vi "DRIVE PID.vi"(9 "SP2:":dbl(slide)=35.294117647058826 min=0.0 max=0.0 scale=0.0..100.0, 10 "SP1:":dbl(slide)=60.7843137254902 min=0.0 max=0.0 scale=0.0..100.0) -> ()   [LabVIEW 2020]
doc: "This example demonstrates how to create a dual PID controller."
uses:
  <vilib>/addons/control/pid/pid.llb/PID (DBL).vi
  <vilib>/addons/control/pid/NI_PID_pid.lvlib
panel:
  in  "derivative time (Td, min) 2":dbl format="%.3f"
  in  "integral time (Ti, min) 2":dbl=0.056 format="%.3f"
  in  "proportional gain (Kc) 2":dbl=50.0 format="%.3f"
  in  "derivative time (Td, min)":dbl=0.001 format="%.3f"
  in  "integral time (Ti, min)":dbl=0.1 format="%.3f"
  in  "proportional gain (Kc)":dbl=50.0 format="%.3f"
  out "MV2:":dbl(slide)=100.0 scale=-100.0..100.0
  out "PV2:":dbl(slide)=19.422100390987225 scale=0.0..100.0
  out "MV1:":dbl(slide)=100.0 scale=-100.0..100.0
  out "PV1:":dbl(slide)=29.253567073551352 scale=0.0..100.0
  in  "Sampling Time dt (s)":dbl=0.05 min=0.001 step=0.01 format="%#.3p"
  in  "Stop":bool
  out "Process Variable and Setpoint":T1(graph)={"initial PV"=29.253567073551352, "SP1:"=60.7843137254902, "initial PV"=19.422100390987225, "SP2:"=35.294117647058826}
  # "Overview: This example demonstrates how to create a dual PID controller.\nInstructions:\n1. Run the VI and observe the Process Variable (PV) following the Setpoint (SP) for both Controllers.\n2. Change the setpoint of one controller and verify that it does not affect the second controller.\n3. Click Stop to stop the VI."
  # "PID Parameters"
  # "Plants Parameters"
  # "Controller 1"
  # "Controller 2"
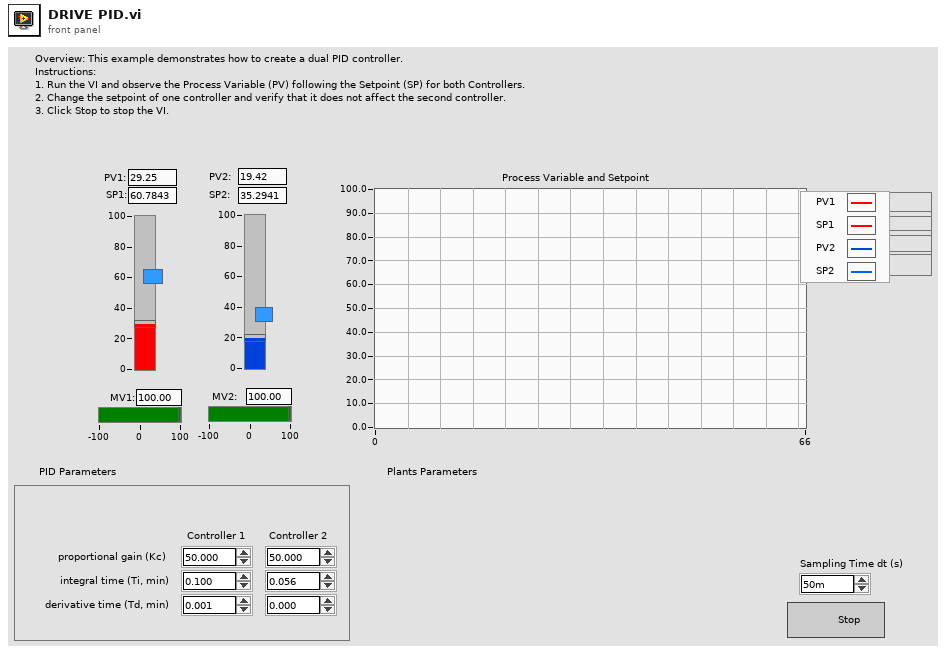
[diagram p1: front panel]
types:
  T1 = cluster{"initial PV":dbl, "SP1:":dbl, "initial PV":dbl, "SP2:":dbl}
  T2 = cluster{"proportional gain (Kc)":dbl, "integral time (Ti, min)":dbl, "derivative time (Td, min)":dbl}
  T3 = cluster{"proportional gain (Kc) 2":dbl, "integral time (Ti, min) 2":dbl, "derivative time (Td, min) 2":dbl}
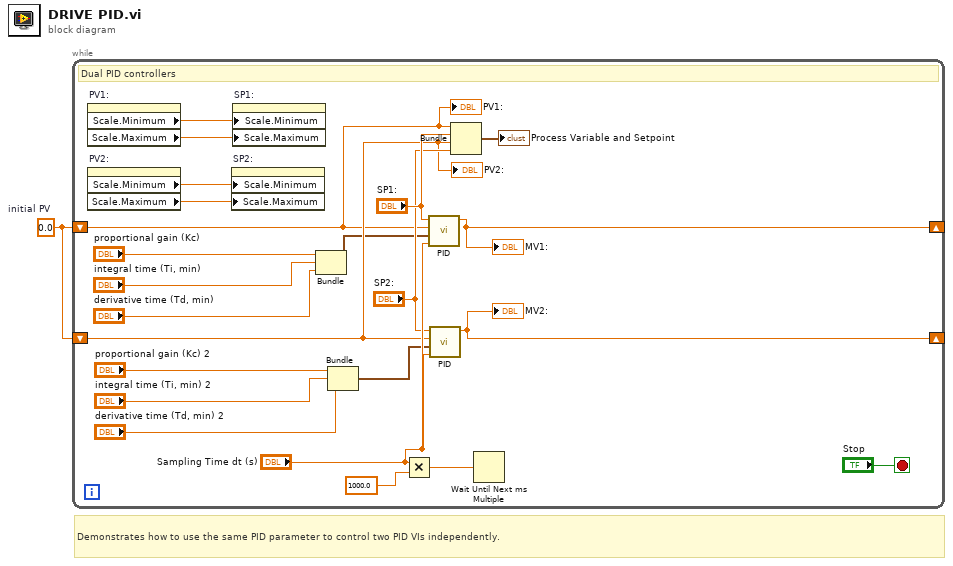
[diagram p0: block diagram]
diagram:
  w1 = 0.0  # initial PV
  # "Demonstrates how to use the same PID parameter to control two PID VIs independently."
  n1 = while {
    shift-left: w1 -> [w12]
    shift-right: [w22] -> _
    shift-right: [w17] -> _
    shift-left: w1 -> [w13]
    stop <- "Stop" stop-if-true
    # "Dual PID controllers"
    n2 = property on="PV1:" class="Slide (strict)"() -> ("Scale.Minimum"=w20:dbl, "Scale.Maximum"=w19:dbl)  [unwired: 2 in, 2 out]
    n3 = property on="PV2:" class="Slide (strict)"() -> ("Scale.Minimum"=w16:dbl, "Scale.Maximum"=w15:dbl)  [unwired: 2 in, 2 out]
    n4 = property on="SP2:" class="Slide (strict)"("Scale.Minimum"=w16, "Scale.Maximum"=w15) -> ()  [unwired: 2 in, 2 out]
    n5 = property on="SP1:" class="Slide (strict)"("Scale.Minimum"=w20, "Scale.Maximum"=w19) -> ()  [unwired: 2 in, 2 out]
    n6 = Bundle("proportional gain (Kc)"="proportional gain (Kc)", "integral time (Ti, min)"="integral time (Ti, min)", "derivative time (Td, min)"="derivative time (Td, min)") -> (w8:T2)  [unwired: 1 in]
    n7 = Bundle("proportional gain (Kc) 2"="proportional gain (Kc) 2", "integral time (Ti, min) 2"="integral time (Ti, min) 2", "derivative time (Td, min) 2"="derivative time (Td, min) 2") -> (w4:T3)  [unwired: 1 in]
    n8 = Multiply(x="Sampling Time dt (s)", y=1000.0) -> (x*y=w3:dbl)
    n9 = call-poly <vilib>:"PID.vi"("dt (s)"="Sampling Time dt (s)", "PID gains"=w8, "process variable"=w12, "setpoint"="SP1:") -> ("output"=w22:dbl)  [unwired: 6 in, 1 out]
    "MV1:" <- w22
    n10 = call-poly <vilib>:"PID.vi"("dt (s)"="Sampling Time dt (s)", "PID gains"=w4, "process variable"=w13, "setpoint"="SP2:") -> ("output"=w17:dbl)  [unwired: 6 in, 1 out]
    "MV2:" <- w17
    n11 = Bundle("initial PV"=w12, "SP1:"="SP1:", "initial PV"=w13, "SP2:"="SP2:") -> (→"Process Variable and Setpoint":T1)  [unwired: 1 in]
    n12 = Wait Until Next ms Multiple(millisecond multiple=w3) -> ()  [unwired: 1 out]
    "PV1:" <- w12
    "PV2:" <- w13
  }
